vi "Stop Core.vi"(10 "final error code":i32, 11 "RDS Local Remote Actor in":refnum<class "RDS Local Remote Actor.lvclass">) -> (3 "RDS Local Remote Actor out":refnum<class "RDS Local Remote Actor.lvclass">)   [LabVIEW 2015, in "RDS Local Remote Actor.lvlib" / "RDS Local Remote Actor.lvclass"]
doc: "(<B>Filename</B>: Actor Framework.lvlib:Actor.lvclass:Stop Core.vi)\n\nDefines what the actor does before it stops. Use the <B>final error code</B> input to determine whether the actor shut down in response to an error.\n\nBy default, this method does nothing. A descendant class may override it to define behavior, such as shutting down any processes the actor initiated in its override of the Actor Core method."
uses:
  RDS Local Remote Actor.lvclass
  RDS Local Remote Actor.lvclass/RDS Local Remote Actor.ctl
  <vilib>/Utility/inputDevices.llb/closeJoystick.vi
  RDS Parent Actor/RDS Parent Actor/RDS Parent Actor.lvclass
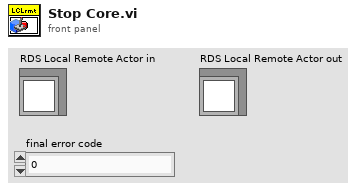
[diagram p1: front panel]
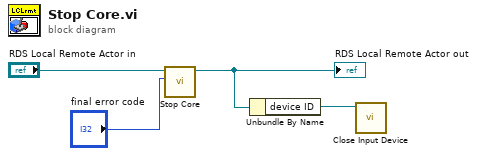
[diagram p0: block diagram]
diagram:
  n1 = call-parent "Stop Core.vi"("final error code"="final error code", "RDS Parent Actor in"="RDS Local Remote Actor in") -> ("RDS Parent Actor out"=w2:refnum<class "RDS Local Remote Actor.lvclass">)  [unwired: 9 in]
  "RDS Local Remote Actor out" <- w2
  n2 = Unbundle By Name(w2) -> ("device ID"=w1:refnum<k1>)
  n3 = call-poly <vilib>:"Close Input Device.vi"("device ID"=w1) -> ()  [unwired: 9 in, 1 out]
